vi "onIncomingMessagingError.vi"(8 "error in (no error)":errorcluster, 10 "model in":refnum<class "IModel.lvclass">, 11 "DisabledState in":refnum<class "DisabledState.lvclass">) -> (0 "error out":errorcluster, 2 "model out":refnum<class "IModel.lvclass">, 3 "DisabledState out":refnum<class "DisabledState.lvclass">)   [LabVIEW 2016, in "States.lvlib" / "DisabledState.lvclass"]
uses:
  DisabledState.lvclass
  IModel/IModel.lvclass
  ts_sallv_sedspectrometer/DataTypes/logevent_SummaryState.ctl
  ts_sallv_sedspectrometer/DataTypes/logevent_DetailedState.ctl
  ComponentTemplateCore/ComponentModel/ComponentModel/InternalSignals/error.vi
  ComponentTemplateCore/ComponentModel/ComponentModel/InternalSignals/InternalSignalsGlobals.lvlib
  ts_sallv_sedspectrometer/SALLV_sedSpectrometer.lvlib
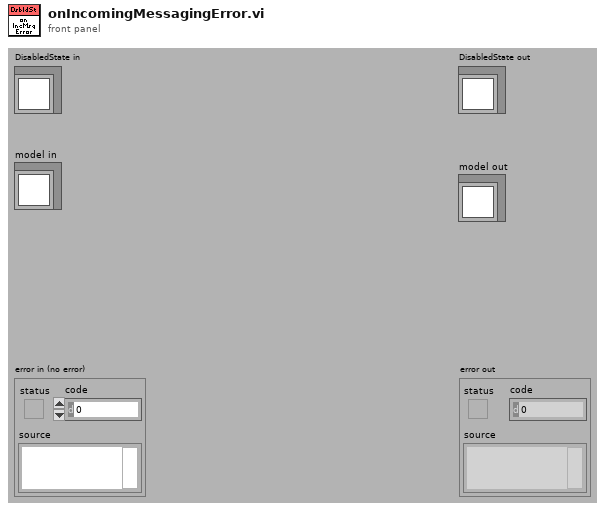
[diagram p1: front panel]
types:
  T1 = typedef "SALLV_sedSpectrometer.lvlib/logevent_DetailedState.ctl" = cluster{"detailedState":enum16{"", "DisabledState", "EnabledState", "FaultState", "OfflineState", "StandbyState"}, "priority":i32}
  T2 = typedef "SALLV_sedSpectrometer.lvlib/logevent_SummaryState.ctl" = cluster{"summaryState":enum16{"", "DisabledState", "EnabledState", "FaultState", "OfflineState", "StandbyState"}, "priority":i32}
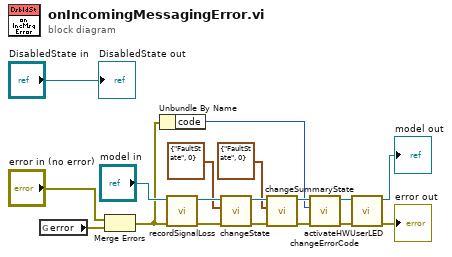
[diagram p0: block diagram]
diagram:
  n1 = global read "error.vi" "error"() -> (w11:errorcluster)
  n2 = Merge Errors("error in (no error)", w11) -> (w4:errorcluster)
  n3 = Unbundle By Name(w4) -> ("code"=w14:i32)
  n4 = call-dynamic "recordSignalLoss.vi"("error in (no error)"=w4, "IModel in"="model in") -> ("error out"=w3:errorcluster, "IModel out"=w5:refnum<class "IModel.lvclass">)  [unwired: 8 in]
  n5 = call-dynamic "changeState.vi"("error in (no error)"=w3, "DetailedState"=T1 {"detailedState"=enum."FaultState", "priority"=0} ("logevent_DetailedState"), "IModel in"=w5) -> ("error out"=w16:errorcluster, "IModel out"=w18:refnum<class "IModel.lvclass">)  [unwired: 7 in]
  n6 = call-dynamic "changeSummaryState.vi"("error in (no error)"=w16, "logevent_SummaryState"=T2 {"summaryState"=enum."FaultState", "priority"=0}, "IModel in"=w18) -> ("error out"=w15:errorcluster, "IModel out"=w17:refnum<class "IModel.lvclass">)  [unwired: 7 in]
  n7 = call-dynamic "changeErrorCode.vi"("error in (no error)"=w15, "error.code"=w14, "IModel in"=w17) -> ("error out"=w8:errorcluster, "IModel out"=w10:refnum<class "IModel.lvclass">)  [unwired: 7 in]
  n8 = call-dynamic "activateHWUserLED.vi"("error in (no error)"=w8, "IModel in"=w10) -> ("error out"=→"error out":errorcluster, "IModel out"=→"model out":refnum<class "IModel.lvclass">)  [unwired: 8 in]
  "DisabledState out" <- "DisabledState in"
